vi "Pincher Controller.vi"(8 "error in":errorcluster) -> ()   [LabVIEW 2017]
doc: "This VI executes continuously carrying out the current operation and responding to updates or new operations. It will often contain the timing or control code that is difficult to place directly in TeleOp. This VI generally opens all sensors and motors and isolates the rest of the robot code from knowing how the operations are carried out."
uses:
  <vilib>/Rock Robotics/WPI/Framework/Completion Status.ctl
  Pincher Setpoints.ctl
  Pincher Operations.ctl
  <vilib>/Rock Robotics/WPI/MotorControl/WPI_MotorControlDeviceRef.ctl
  <vilib>/Rock Robotics/WPI/MotorControl/WPI_MotorControlType.ctl
  <vilib>/Rock Robotics/SystemInterfaces/DIO/FPGA_DIOPWMChannel.ctl
  <vilib>/Rock Robotics/WPI/PWM/WPI_PWMDeadband.ctl
  <vilib>/Rock Robotics/SystemInterfaces/DIO/FPGA_DIOChannel.ctl
  <vilib>/Rock Robotics/WPI/ThirdParty/Phoenix-LabVIEW/Motor Controller/Controls/CTRE_Phoenix_MotorControl_ControlMode.ctl
  Framework/Robot Global Data.vi
  <vilib>/Rock Robotics/WPI/ThirdParty/Phoenix-LabVIEW/Motor Controller/Get/CTRE_Phoenix_MotorController_GetVoltage.vi
  <vilib>/Rock Robotics/WPI/ThirdParty/Phoenix-LabVIEW/Motor Controller/Get/CTRE_Phoenix_MotorController_GetOutputCurrent_Enhanced.vi
  Support Code/Global Constants.vi
  <vilib>/Rock Robotics/Network Tables/NT Write Boolean.vi
panel:
  out "Pinch Output":dbl(graph)
  out "Pinch Output 2":dbl
  out "Pinch Current":dbl(graph)=0.125
  out "Pinch Current 2":dbl=0.125
  in  "Pincher P":dbl=0.3 format="%#_13g"
  in  "Pincher F":dbl format="%#_13g"
  in  "Interactive Values":T1
  out "Current\nCmd":string
  in  "Buttons":cluster{"Execute Cmd":bool, "Abort Cmd":bool}
  out "Command Timing":cluster{"Start Time (ms)":u32, "Iterations":i32}
  out "Status":T3
  # "Tip: It may be helpful to observe inputs and sensor values.\nYou may also want to display tuning or debugging controls."
  # "Interactive Command: You may fill in the settings for a command\nand schedule it with the Execute button. You can observe and abort\nany command while fine tuning the code for the controller."
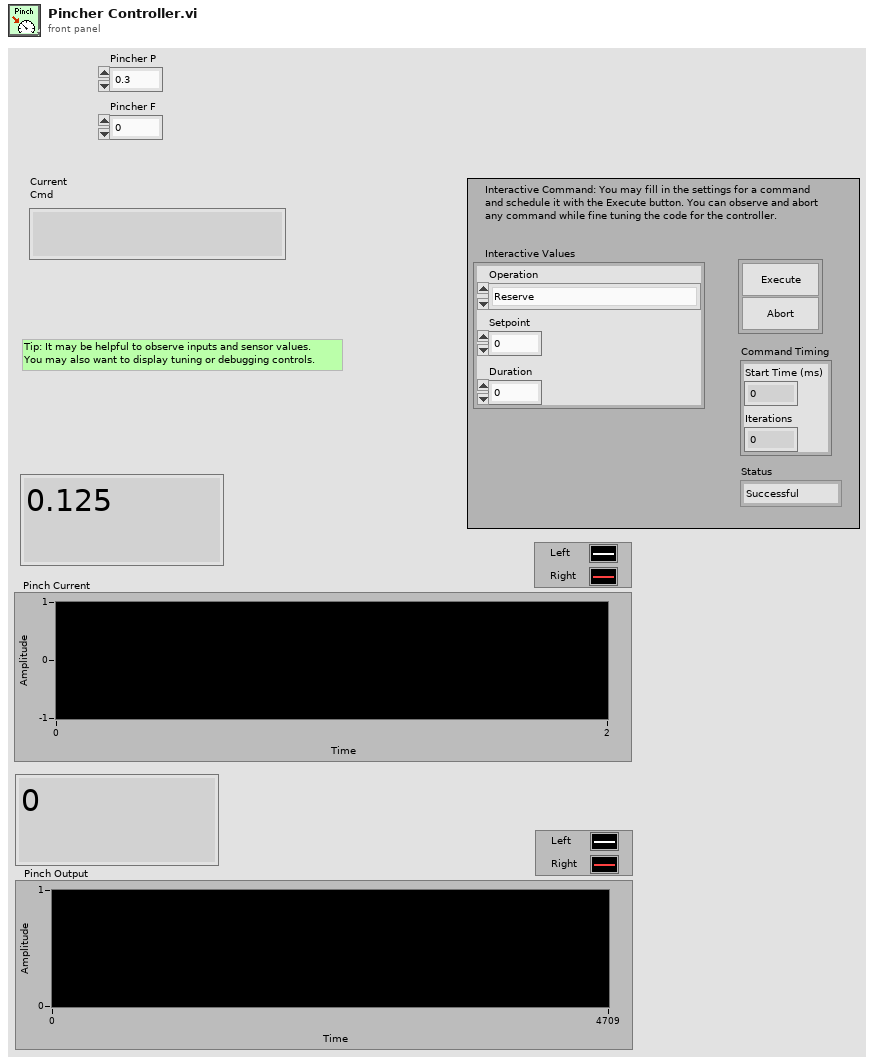
[diagram p1: front panel]
types:
  T1 = typedef "Pincher Setpoints.ctl" = cluster{"Operation":T2, "Setpoint":dbl, "Duration":dbl}
  T2 = typedef "Pincher Operations.ctl" = enum16{"Reserve", "Read Current", "Immediate", "Hold Amp", "Hold Amp for duration"}
  T3 = typedef "Completion Status.ctl" = enum16{"Successful", "Aborted", "Incomplete"}
  T4 = typedef "WPI_MotorControlDeviceRef.ctl" = cluster{"DeviceStatus":errorcluster, "Type":T5, "PWM":cluster{"PWM Channel":T6, "DeadBand":T7}, "CAN":cluster{"Device Number":u8, "SetOutput VI Ref":variant, "GetOutput VI Ref":variant, "Enable VI Ref":variant, "Disable VI Ref":variant, "Data":variant}, "Invert":bool, "DIO PWM":cluster{"PWM \"Enable\" Channel":T6, "DIOChannel":T8, "PWM Rate":dbl}}
  T5 = typedef "WPI_MotorControlType.ctl" = enum16{"PWM", "CAN", "DIO PWM"}
  T6 = typedef "FPGA_DIOPWMChannel.ctl" = enum8{"PWM 0", "PWM 1", "PWM 2", "PWM 3", "PWM 4", "PWM 5", "PWM 6", "PWM 7", "PWM 8", "PWM 9", "PWM MXP 0", "PWM MXP 1", "PWM MXP 2", "PWM MXP 3", "PWM MXP 4", "PWM MXP 5", "PWM MXP 6", "PWM MXP 7", "PWM MXP 8", "PWM MXP 9", "Invalid"}
  T7 = typedef "WPI_PWMDeadband.ctl" = cluster{"Name":string, "maxPositivePwm":i32, "minPositivePwm":i32, "centerPwm":i32, "maxNegativePwm":i32, "minNegativePwm":i32, "angularRange":u16}
  T8 = typedef "FPGA_DIOChannel.ctl" = enum8{"DIO 0", "DIO 1", "DIO 2", "DIO 3", "DIO 4", "DIO 5", "DIO 6", "DIO 7", "DIO 8", "DIO 9", "DIO MXP 0", "DIO MXP 1", "DIO MXP 2", "DIO MXP 3", "DIO MXP 4", "DIO MXP 5", "DIO MXP 6", "DIO MXP 7", "DIO MXP 8", "DIO MXP 9", "DIO MXP 10", "DIO MXP 11", "DIO MXP 12", "DIO MXP 13", "DIO MXP 14", "DIO MXP 15", "SPI Port CS1", "SPI Port CS2", "SPI Port CS3", "SPI Port MISO", "SPI Port MOSI", "Invalid"}
  T9 = typedef "Command Status Info.ctl" = cluster{"Name":string, "Status":T3, "notifier out":T10}
  T10 = typedef "Completion Notifier.ctl" = refnum<notifier>
  T11 = cluster{"Current Command":T1, "Command Timing":cluster{"Start Time (ms)":u32, "Iterations":i32}, "Command Arguments":cluster{"Command Info":T9, "Description":string, "Default Command":T1, "queue out":refnum<queue>, "Subsystem Name":string}}
  T12 = typedef "CTRE_Phoenix_MotorControl_ControlMode.ctl" = u16
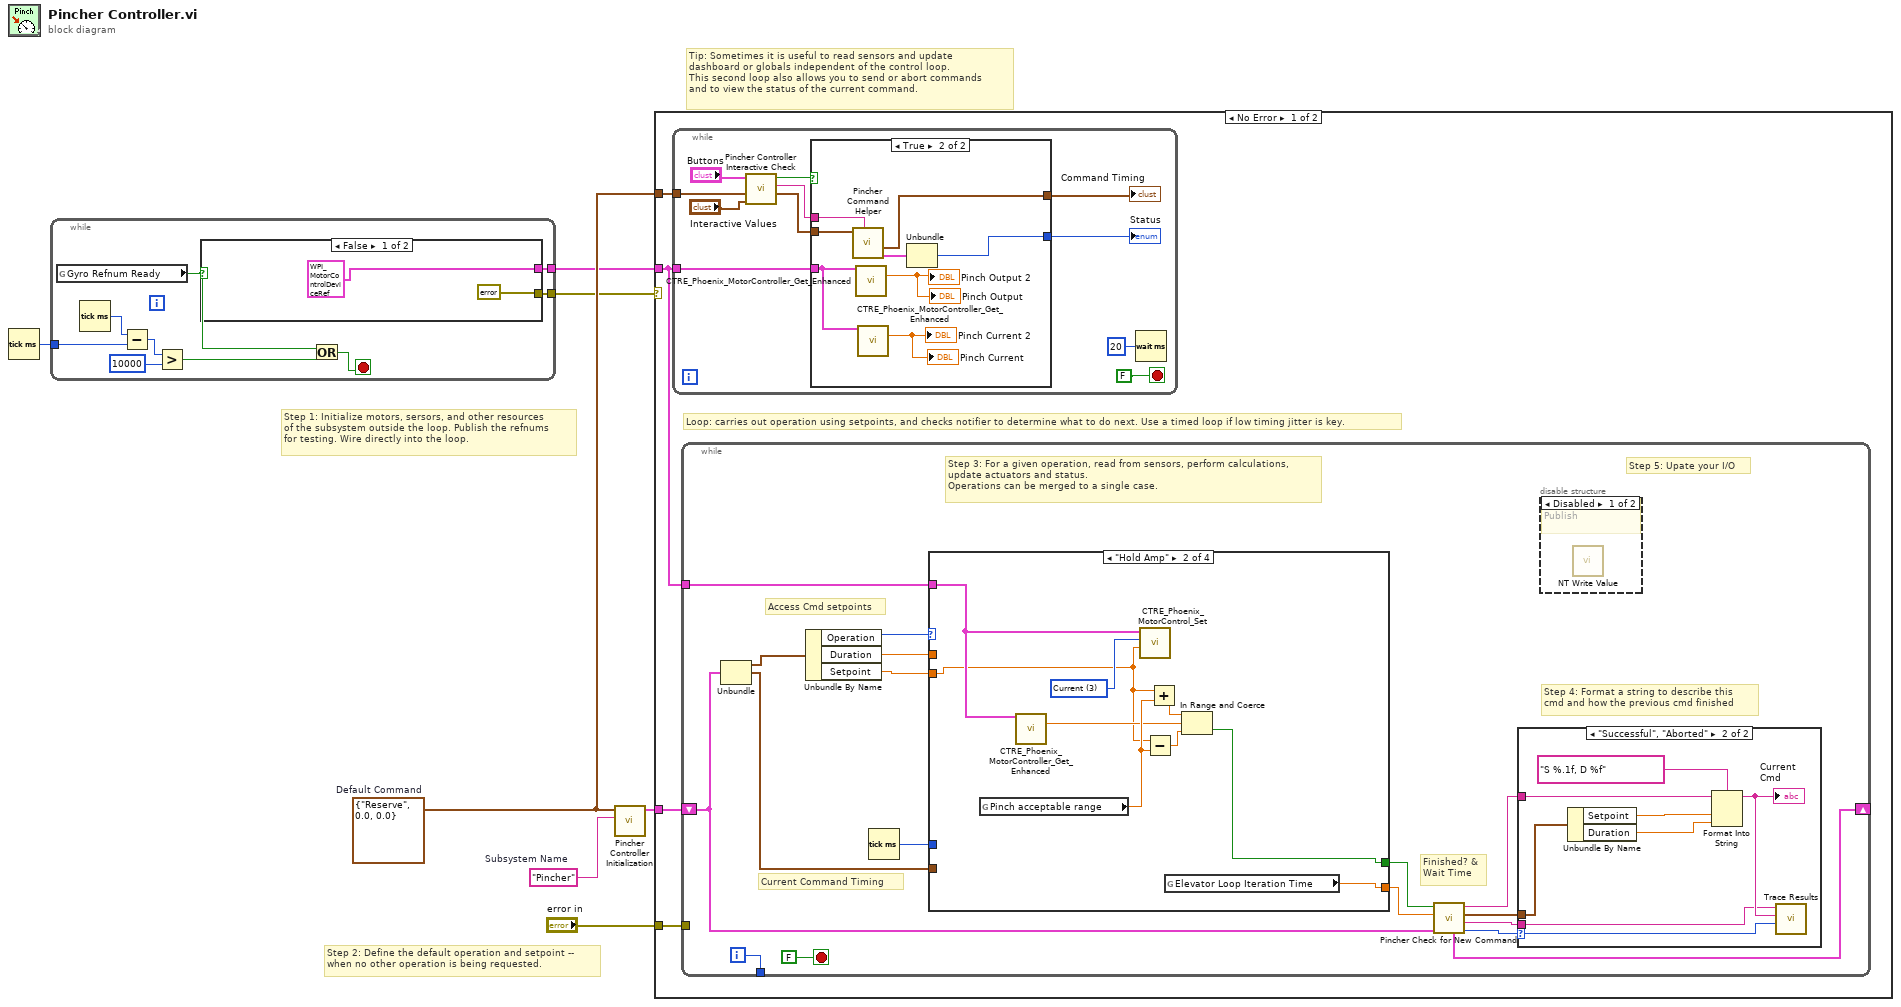
[diagram p0: block diagram]
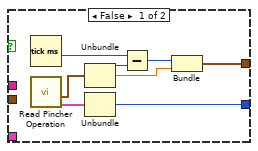
[diagram p2: hidden frame]
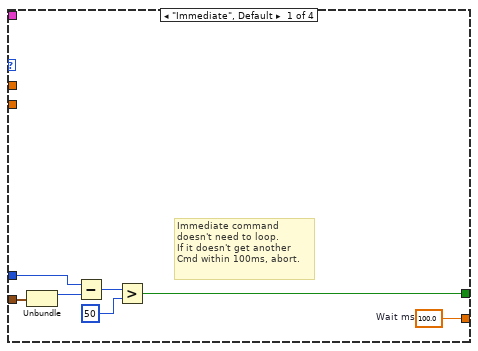
[diagram p5: hidden frame]
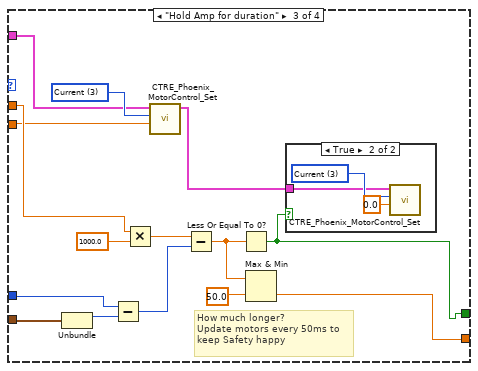
[diagram p6: hidden frame]
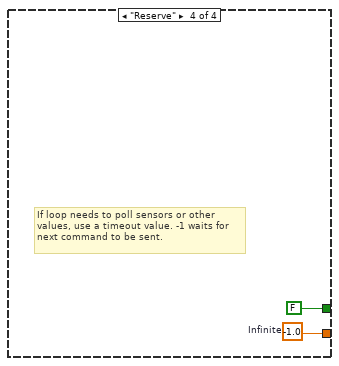
[diagram p8: hidden frame]
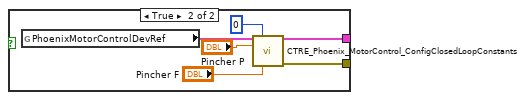
[diagram p10: hidden frame]
diagram:
  w4 = T1 {"Operation"=enum."Reserve", "Setpoint"=0.0, "Duration"=0.0}  # Default Command
  w5 = "Pincher"  # Subsystem Name
  # "Tip: Sometimes it is useful to read sensors and update\ndashboard or globals independent of the control loop.\nThis second loop also allows you to send or abort commands\nand to view the status of the current command."
  # "Step 2: Define the default operation and setpoint --\nwhen no other operation is being requested."
  # "Step 1: Initialize motors, sersors, and other resources\nof the subsystem outside the loop. Publish the refnums\nfor testing. Wire directly into the loop."
  n1 = Tick Count (ms)() -> (millisecond timer value=w3:u32)
  n2 = while {
    tunnel: [w16] -> w2
    tunnel: w3 -> [w13]
    tunnel: [w8] -> w1
    stop <- w15 stop-if-true
    n3 = global read "Robot Global Data.vi" "Gyro Refnum Ready"() -> (w14:bool)
    n4 = Tick Count (ms)() -> (millisecond timer value=w12:u32)
    n5 = Subtract(x=w12, y=w13) -> (x-y=w11:u32)
    n6 = Greater?(x=w11, y=u32 10000) -> (0:w9:bool)
    n7 = case shown="False" w14 {
      tunnel: [T4 {"DeviceStatus"={"status"=FALSE, "code"=0, "source"=""}, "Type"=enum."PWM", "PWM"={"PWM Channel"=enum."Invalid", "DeadBand"={"Name"="", "maxPositivePwm"=0, "minPositivePwm"=0, "centerPwm"=0, "maxNegativePwm"=0, "minNegativePwm"=0, "angularRange"=0}}, "CAN"={"Device Number"=0, "SetOutput VI Ref"=variant, "GetOutput VI Ref"=variant, "Enable VI Ref"=variant, "Disable VI Ref"=variant, "Data"=variant}, "Invert"=FALSE, "DIO PWM"={"PWM \"Enable\" Channel"=enum."Invalid", "DIOChannel"=enum."Invalid", "PWM Rate"=0.0}} ("CAN Talon SRX Ref") w21] -> w16
      tunnel: [errorcluster {"status"=TRUE, "code"=0, "source"=""} ("error out") w19] -> w8
      frame False {
      }
      frame True {
        n8 = global read "Robot Global Data.vi" "PhoenixMotorControlDevRef"() -> (w24:T4)
        n9 = call <vilib>:"CTRE_Phoenix_MotorControl_ConfigClosedLoopConstants.vi"("PhoenixMotorControlDevRef"=w24, "slotIdx"=0, "P"="Pincher P", "F"="Pincher F") -> ("PhoenixMotorControlDevRef"=w21:T4, "error out"=w19:errorcluster)  [unwired: 10 in]
      }
    }
    n10 = Or(x=w14, y=w9) -> (x .or. y?=w15:bool)
  }
  n11 = call "Pincher Controller Initialization.vi"("Subsystem Name"=w5, "Default Command"=w4) -> ("Current Command"=w6:T11)  [unwired: 9 in]
  n12 = case shown="No Error" w1 {
    tunnel: "error in" -> [w28 _]
    tunnel: w6 -> [w27 _]
    tunnel: w4 -> [w26 _]
    tunnel: w2 -> [w25 _]
    frame No Error {
      # "Loop: carries out operation using setpoints, and checks notifier to determine what to do next. Use a timed loop if low timing jitter is key."
      n13 = while {
        tunnel: w26 -> [w36]
        tunnel: w25 -> [w29]
        stop <- FALSE stop-if-true
        n14 = call "Pincher Controller Interactive Check.vi"("Interactive Command in"="Interactive Values", "Default Command"=w36, "Buttons"="Buttons") -> ("Interactive Command out"=w33:T1, "Trace String"=w34:string, "Schedule"=w35:bool)  [unwired: 6 in]
        n15 = case shown="True" w35 {
          tunnel: [w47 w55] -> w32
          tunnel: w33 -> [_ w53]
          tunnel: [w43 w51] -> w31
          tunnel: w34 -> [_ w54]
          tunnel: w29 -> [_ w48]
          frame False {
            n16 = Tick Count (ms)() -> (millisecond timer value=w42:u32)
            n17 = call "Read Pincher Operation.vi"() -> ("Command Info"=w40:T9, "SubSystem Data"=w41:T1)  [unwired: 9 in, 1 out]
            n18 = Unbundle(w41) -> ("Operation"=w46:T2, "Setpoint"=w44:dbl)  [unwired: 1 out]
            n19 = Unbundle(w40) -> ("Status"=w47:T3)  [unwired: 2 out]
            n20 = Subtract(x=w42, y=w46) -> (x-y=w45:u32)
            n21 = Bundle(w45, "Setpoint"=w44) -> (w43:cluster{u32, "Setpoint":dbl})  [unwired: 1 in]
          }
          frame True {
            n22 = call "Pincher Command Helper.vi"("Description"=w54, "SubSystem Data"=w53) -> ("Command Info Out"=w52:T9, "Command Timing"=w51:cluster{"Start Time (ms)":u32, "Iterations":i32})  [unwired: 7 in, 1 out]
            n23 = call-poly <vilib>:"CTRE_Phoenix_MotorController_Get_Enhanced.vi"("PhoenixMotorControlDevRef"=w48) -> ("Percent Output"=→"Pinch Output 2" →"Pinch Output":dbl)  [unwired: 10 in, 4 out]
            n24 = call-poly <vilib>:"CTRE_Phoenix_MotorController_Get_Enhanced.vi"("PhoenixMotorControlDevRef"=w48) -> ("Output Current"=→"Pinch Current 2" →"Pinch Current":dbl)  [unwired: 12 in, 2 out]
            n25 = Unbundle(w52) -> ("Status"=w55:T3)  [unwired: 2 out]
          }
        }
        "Status" <- w32
        "Command Timing" <- w31
        n26 = Wait (ms)(milliseconds to wait=u32 20) -> ()  [unwired: 1 out]
      }
      n27 = while {
        shift-right: [w64] -> _
        shift-left: w27 -> [w57]
        tunnel: [w71] -> _
        tunnel: w28 -> [_]
        tunnel: w25 -> [w56]
        i -> [w71]
        stop <- FALSE stop-if-true
        # "Step 5: Upate your I/O"
        # "Step 4: Format a string to describe this\ncmd and how the previous cmd finished"
        # "Current Command Timing"
        # "Access Cmd setpoints"
        # "Finished? &\nWait Time"
        # "Step 3: For a given operation, read from sensors, perform calculations,\nupdate actuators and status.\nOperations can be merged to a single case."
        n28 = Unbundle(w57) -> ("Current Command"=w70:T1, "Command Timing"=w66:cluster{"Start Time (ms)":u32, "Iterations":i32})  [unwired: 1 out]
        n29 = Unbundle By Name(w70) -> ("Operation"=w69:T2, "Duration"=w68:dbl, "Setpoint"=w65:dbl)
        n30 = Tick Count (ms)() -> (millisecond timer value=w67:u32)
        n31 = case shown="\"Hold Amp\"" w69 {
          tunnel: [w87 w90 w98 w116] -> w62
          tunnel: [w81 w91 w99 FALSE ("ignore previous (F)")] -> w63
          tunnel: w66 -> [w83 _ w101 _]
          tunnel: w68 -> [_ _ w100 _]
          tunnel: w67 -> [w82 _ w102 _]
          tunnel: w65 -> [_ w88 w97 _]
          tunnel: w56 -> [_ w89 w103 _]
          frame "Immediate", Default {
            w87 = 100.0  # Wait ms
            # "Immediate command\ndoesn't need to loop.\nIf it doesn't get another\nCmd within 100ms, abort."
            n32 = Unbundle(w83) -> ("Start Time (ms)"=w86:u32)  [unwired: 1 out]
            n33 = Subtract(x=w82, y=w86) -> (x-y=w85:u32)
            n34 = Greater?(x=w85, y=u8 50 ("Left Motor")) -> (0:w81:bool)
          }
          frame "Hold Amp" {
            w96 = T12 3 items=["PercentOutput"=0, "Position"=1, "Velocity"=2, "Current"=3, "Follower"=5, "MotionProfile"=6, "MotionMagic"=7, "MotionMagicArc"=8, "MotionProfileArc"=10, "Disabled"=15] ("Control Mode")
            n35 = global read "Global Constants.vi" "Pinch acceptable range"() -> (w94:dbl)
            n36 = call-poly <vilib>:"CTRE_Phoenix_MotorController_Get_Enhanced.vi"("PhoenixMotorControlDevRef"=w89) -> ("Output Current"=w92:dbl)  [unwired: 12 in, 2 out]
            n37 = call <vilib>:"CTRE_Phoenix_MotorControl_Set.vi"("Output"=w88, "Control Mode"=w96, "PhoenixMotorControlDevRef"=w89) -> ()  [unwired: 7 in, 2 out]
            n38 = Subtract(x=w88, y=w94) -> (x-y=w95:dbl)
            n39 = Add(x=w88, y=w94) -> (x+y=w93:dbl)
            n40 = global read "Global Constants.vi" "Elevator Loop Iteration Time"() -> (w90:dbl)
            n41 = In Range and Coerce(upper limit=w93, x=w92, lower limit=w95) -> (In Range?=w91:bool)  [unwired: 1 out]
          }
          frame "Hold Amp for duration" {
            w105 = T12 3 items=["PercentOutput"=0, "Position"=1, "Velocity"=2, "Current"=3, "Follower"=5, "MotionProfile"=6, "MotionMagic"=7, "MotionMagicArc"=8, "MotionProfileArc"=10, "Disabled"=15] ("Control Mode")
            # "How much longer?\nUpdate motors every 50ms to\nkeep Safety happy"
            n42 = Unbundle(w101) -> ("Start Time (ms)"=w108:u32)  [unwired: 1 out]
            n43 = Subtract(x=w102, y=w108) -> (x-y=w111:u32)
            n44 = Multiply(x=w100, y=1000.0) -> (x*y=w110:dbl)
            n45 = call <vilib>:"CTRE_Phoenix_MotorControl_Set.vi"("Output"=w97, "Control Mode"=w105, "PhoenixMotorControlDevRef"=w103) -> ("PhoenixMotorControlDevRef"=w104:T4)  [unwired: 7 in, 1 out]
            n46 = Subtract(x=w110, y=w111) -> (x-y=w107:dbl)
            n47 = Less Or Equal To 0?(x=w107) -> (x <= 0?=w99:bool)
            n48 = Max & Min(x=w107, y=50.0) -> (min(x,y)=w98:dbl)  [unwired: 1 out]
            n49 = case shown="True" w99 {
              tunnel: w104 -> [_ w113]
              frame False {
              }
              frame True {
                w114 = T12 3 items=["PercentOutput"=0, "Position"=1, "Velocity"=2, "Current"=3, "Follower"=5, "MotionProfile"=6, "MotionMagic"=7, "MotionMagicArc"=8, "MotionProfileArc"=10, "Disabled"=15] ("Control Mode")
                n50 = call <vilib>:"CTRE_Phoenix_MotorControl_Set.vi"("Output"=0.0, "Control Mode"=w114, "PhoenixMotorControlDevRef"=w113) -> ()  [unwired: 7 in, 2 out]
              }
            }
          }
          frame "Reserve" {
            w116 = -1.0  # Infinite
            # "If loop needs to poll sensors or other\nvalues, use a timeout value. -1 waits for\nnext command to be sent."
          }
        }
        n51 = call "Pincher Check for New Command.vi"("Current Command"=w57, "Wait time (ms)"=w62, "Finished?"=w63) -> ("Completion"=w58:T3, "Subsystem Name"=w59:string, "Current Command"=w60:T1, "Initial Trace String"=w61:string, "NextCommand"=w64:T11)  [unwired: 4 in]
        n52 = case shown="\"Successful\", \"Aborted\"" w58 {
          selector: w58 -> [_ w80]
          tunnel: w61 -> [_ w76]
          tunnel: w60 -> [_ w77]
          tunnel: w59 -> [_ w73]
          frame "Incomplete", Default {
            # "Continuing current command"
          }
          frame "Successful", "Aborted" {
            # "Report and setup for next command"
            n53 = Unbundle By Name(w77) -> ("Setpoint"=w79:dbl, "Duration"=w74:dbl)
            n54 = Format Into String(format string="S %.1f, D %f", initial string=w76, w79, w74) -> (resulting string=w75:string)  [unwired: 1 in, 1 out]
            "Current\nCmd" <- w75
            n55 = call <vilib>:"Trace Results.vi"("Status of previous command"=w80, "Description"=w75, "Subsystem"=w73) -> ()  [unwired: 9 in]
          }
        }
        n56 = disable-structure shown="Disabled" {
          frame Disabled {
            # "Publish"
            n57 = call-poly <vilib>:"NT Write Value.vi"() -> ()  [unwired: 11 in, 1 out]
          }
          frame Enabled {
          }
        }
      }
    }
    frame Error {
    }
  }
